vi "aula1.vi"() -> ()   [LabVIEW 2020]
panel:
  out "element":dbl
  in  "Numeric":i32
  out "Meter":dbl(knob) scale=0.0..50.0
  out "elemento":i32
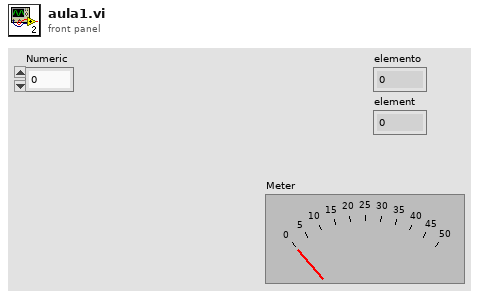
[diagram p1: front panel]
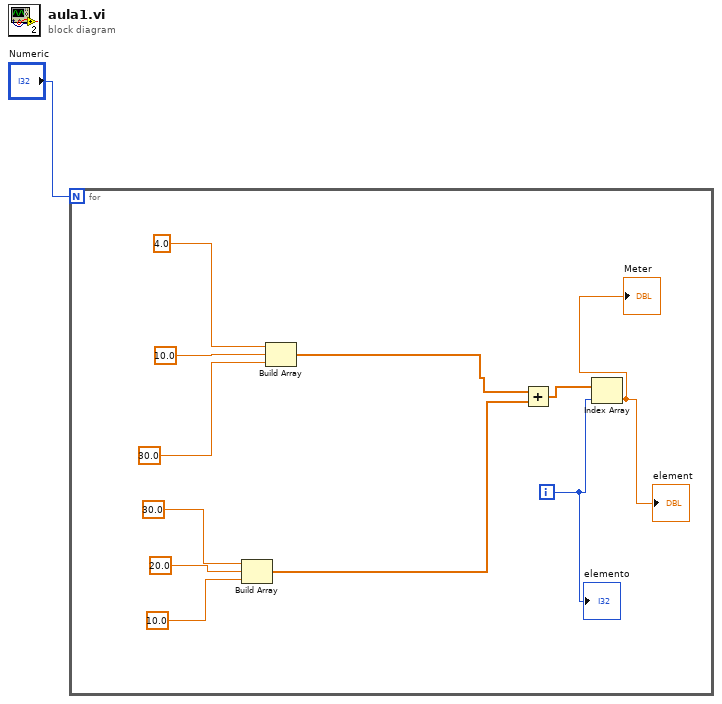
[diagram p0: block diagram]
diagram:
  n1 = for {
    N: "Numeric" -> [_]
    i -> [w3]
    n2 = Build Array(30.0 ("element"), 20.0 ("element"), 10.0 ("element")) -> (w5:dbl[])
    n3 = Build Array(4.0 ("element"), 10.0 ("element"), 30.0 ("element")) -> (w6:dbl[])
    n4 = Add(x=w6, y=w5) -> (x+y=w4:dbl[])
    n5 = Index Array(array=w4, index=w3) -> (element=→"Meter" →"element":dbl)
    "elemento" <- w3
  }
